vi "p-p0 and normaiize_new.vi"(4 "P1 power":dbl[](array[numeric]), 5 "P1 wavelength":dbl[](array[numeric]), 6 "P0 power":dbl[](array[numeric]), 7 "P0 wavelength":dbl[](array[numeric])) -> (0 "SPR efficiency":dbl, 1 "SPR wave length(nm)":dbl, 3 "normallize power":dbl[](array[numeric]))   [LabVIEW 2019]
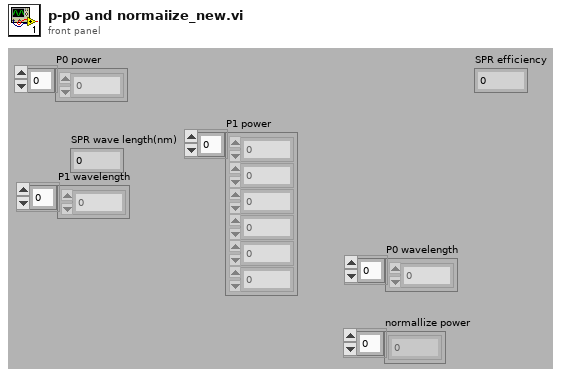
[diagram p1: front panel]
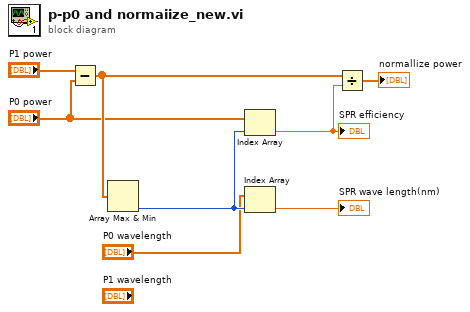
[diagram p0: block diagram]
diagram:
  n1 = Subtract(x="P1 power", y="P0 power") -> (x-y=w6:dbl[])
  n2 = Array Max & Min(array=w6) -> (min index (indices)=w5:i32)  [unwired: 3 out]
  n3 = Index Array "Index Array"(array="P0 power", index=w5) -> (element=w3:dbl)
  "SPR efficiency" <- w3
  n4 = Index Array "Index Array"(array="P0 wavelength", index=w5) -> (element=→"SPR wave length(nm)":dbl)
  n5 = Divide(x=w6, y=w3) -> (x/y=→"normallize power":dbl[])
